vi "Evaluate Fitness.vi"(8 "error in":errorcluster, 10 "IChromosome Target in":refnum<class "IChromosome.lvclass">, 11 "Solution in":refnum<class "Solution.lvclass">) -> (0 "error out":errorcluster, 3 "Solution out":refnum<class "Solution.lvclass">)   [LabVIEW 2016, in "Solution.lvclass"]
uses:
  Solution.lvclass
  C:/Users/J51654/My Projects/Evolutionary Programming/GA Framework/IChromosome/IChromosome.lvclass
  IChromosome/IChromosome.lvclass
  Gene/Bit.lvclass
  IChromosome/IChromosome.lvclass/IChromosome.ctl
  Gene/Bit.lvclass/Bit.ctl
  IGene/IGene.lvclass
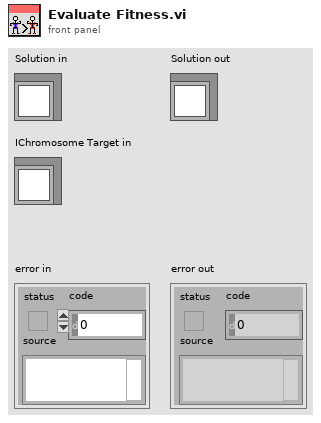
[diagram p1: front panel]
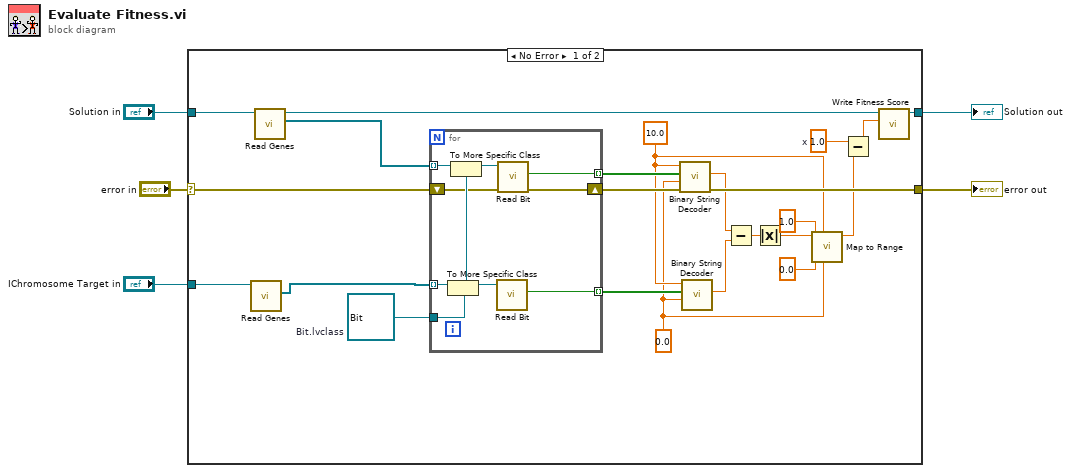
[diagram p0: block diagram]
diagram:
  n1 = case shown="No Error" "error in" {
    selector: "error in" -> [w24 w38]
    tunnel: [w27 w38] -> w4
    tunnel: [w20 w37] -> w2
    tunnel: "Solution in" -> [w26 w37]
    tunnel: "IChromosome Target in" -> [w23 _]
    frame No Error {
      w7 = 1.0  # x
      w11 = 0.0 ("X_L (0.0)")
      w12 = 10.0 ("X_U (1.0)")
      w19 = refnum<class "Bit.lvclass"> refnum  # Bit.lvclass
      n2 = call "Read Genes.vi"("IChromosome in"=w23) -> ("Genes"=w22:refnum<class "IGene.lvclass">[])  [unwired: 8 in, 2 out]
      n3 = call "Read Genes.vi"("IChromosome in"=w26) -> ("Genes"=w25:refnum<class "IGene.lvclass">[], "IChromosome out"=w21:refnum<class "Solution.lvclass">)  [unwired: 8 in, 1 out]
      n4 = for {
        tunnel: w25 -> [w36] mode=indexing
        shift-right: [w28] -> w27
        shift-left: w24 -> [w32]
        tunnel: w22 -> [w35] mode=indexing
        tunnel: w19 -> [w34]
        tunnel: [w30] -> w17 mode=indexing
        tunnel: [w29] -> w18 mode=indexing
        n5 = To More Specific Class(target class=w34, reference=w35) -> (specific class reference=w31:refnum<class "Bit.lvclass">)  [unwired: 1 in, 1 out]
        n6 = To More Specific Class(target class=w34, reference=w36) -> (specific class reference=w33:refnum<class "Bit.lvclass">)  [unwired: 1 in, 1 out]
        n7 = call "Read Bit.vi"("Bit in"=w31) -> ("Bit"=w29:bool)  [unwired: 8 in, 2 out]
        n8 = call "Read Bit.vi"("error in (no error)"=w32, "Bit in"=w33) -> ("error out"=w28:errorcluster, "Bit"=w30:bool)  [unwired: 7 in, 1 out]
      }
      n9 = call "Binary String Decoder.vi"("X_L (0.0)"=w11, "Binary String (LSb[0] - MSb[n-1])"=w17, "X_U (1.0)"=w12) -> ("x"=w16:dbl)  [unwired: 8 in]
      n10 = call "Binary String Decoder.vi"("X_L (0.0)"=w11, "Binary String (LSb[0] - MSb[n-1])"=w18, "X_U (1.0)"=w12) -> ("x"=w15:dbl)  [unwired: 8 in]
      n11 = Subtract(x=w16, y=w15) -> (x-y=w14:dbl)
      n12 = Absolute Value(x=w14) -> (abs(x)=w13:dbl)
      n13 = call "Map to Range.vi"("Value Min"=w11, "Value Max"=w12, "Scale Min"=0.0, "Scale Max"=1.0, "Value"=w13) -> ("Mapped Value"=w8:dbl)  [unwired: 6 in]
      n14 = Subtract(x=w7, y=w8) -> (x-y=w6:dbl)
      n15 = call "Write Fitness Score.vi"("Fitness Score"=w6, "IChromosome in"=w21) -> ("IChromosome out"=w20:refnum<class "Solution.lvclass">)  [unwired: 8 in, 1 out]
    }
    frame Error {
    }
  }
  "error out" <- w4
  "Solution out" <- w2
